vi "json_cluster.vi"(7 "indent level":i32, 10 "array of JSON values":string[](array[string]), 11 "array of element names":string[](array[string])) -> (3 "indented string":string)   [LabVIEW 2013, in "Caraya.lvlib" / "Test Result.lvclass"]
uses:
  Test Result.lvclass
  <vilib>/Utility/error.llb/whitespace.ctl
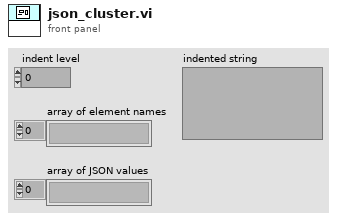
[diagram p1: front panel]
types:
  T1 = typedef "whitespace.ctl" = u16
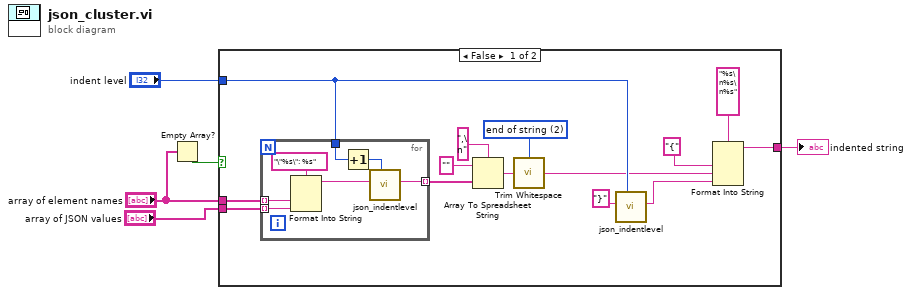
[diagram p0: block diagram]
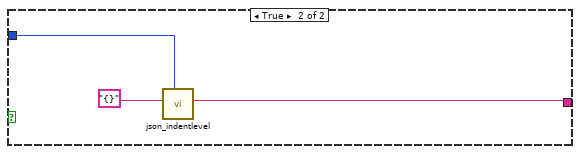
[diagram p2: hidden frame]
diagram:
  n1 = Empty Array?(array="array of element names") -> (empty?=w1:bool)
  n2 = case shown="False" w1 {
    tunnel: "indent level" -> [w19 w29]
    tunnel: "array of JSON values" -> [w12 _]
    tunnel: [w9 w27] -> w3
    tunnel: "array of element names" -> [w7 _]
    frame False {
      w15 = T1 2 items=["both", "start of string", "end of string"] ("location (both)")
      n3 = for {
        tunnel: w7 -> [w26] mode=indexing
        tunnel: w12 -> [w25] mode=indexing
        tunnel: [w22] -> w17 mode=indexing
        tunnel: w19 -> [w21]
        n4 = Format Into String(format string="\"%s\": %s" ("string"), w26, w25) -> (resulting string=w23:string)  [unwired: 2 in, 1 out]
        n5 = Increment(x=w21) -> (x+1=w20:i32)
        n6 = call "json_indentlevel.vi"("indent level"=w20, "string"=w23) -> ("indented string"=w22:string)  [unwired: 9 in]
      }
      n7 = Array To Spreadsheet String(delimiter (Tab)=",\n", array=w17, 3:"" ("format string")) -> (spreadsheet string=w16:string)
      n8 = call <vilib>:"Trim Whitespace.vi"("string"=w16, "location (both)"=w15) -> ("trimmed string"=w18:string)
      n9 = call "json_indentlevel.vi"("indent level"=w19, "string"="}") -> ("indented string"=w11:string)  [unwired: 9 in]
      n10 = Format Into String(format string="%s\n%s\n%s", "{" ("string"), w18, w11) -> (resulting string=w9:string)  [unwired: 2 in, 1 out]
    }
    frame True {
      n11 = call "json_indentlevel.vi"("indent level"=w29, "string"="{}") -> ("indented string"=w27:string)  [unwired: 9 in]
    }
  }
  "indented string" <- w3
